vi "Close Panel TK.vi"(8 "error in (no error)":errorcluster, 11 "VI name":string) -> (0 "error out":errorcluster)   [LabVIEW 2024]
doc: "You can use this VI to close the panel of a specified VI. If the VI is running, it will be aborted."
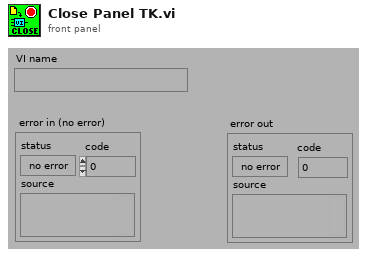
[diagram p1: front panel]
types:
  T1 = enum32{"Bad", "Idle", "Run top level", "Running"}
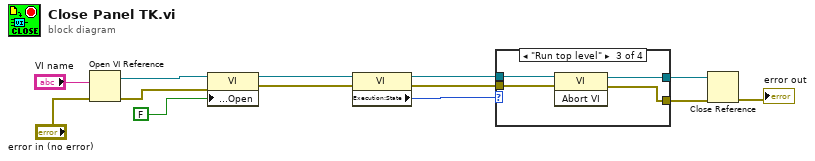
[diagram p0: block diagram]
diagram:
  n1 = Open VI Reference(vi path="VI name", error in (no error)="error in (no error)") -> (vi reference=w3:refnum<vi>, error out=w2:errorcluster)  [unwired: 4 in]
  n2 = property class="VI"(reference=w3, error in=w2, "Front Panel Window:Open"=FALSE ("FPWindOpen")) -> (reference out=w7:refnum<vi>, error out=w8:errorcluster)
  n3 = property class="VI"(reference=w7, error in=w8) -> (reference out=w10:refnum<vi>, error out=w5:errorcluster, "Execution:State"=w4:T1)
  n4 = case shown="\"Run top level\"" w4 {
    tunnel: w5 -> [w15 w17 w20 w23]
    tunnel: [w15 w17 w18 w23] -> w9
    tunnel: w10 -> [w14 w16 w21 w22]
    tunnel: [w14 w16 w19 w22] -> w11
    frame "Bad", Default {
    }
    frame "Idle" {
    }
    frame "Run top level" {
      n5 = invoke class="VI" method="Abort VI"(reference=w21, error in=w20) -> (reference out=w19:refnum<vi>, error out=w18:errorcluster)  [unwired: 1 in, 1 out]
    }
    frame "Running" {
    }
  }
  n6 = Close Reference(reference=w11, error in (no error)=w9) -> (error out=→"error out":errorcluster)
